vi "LIA Select Decimator.vi"(8 "error in (no error)":errorcluster, 9 "lock-in.decimator 0":enum16{"CIC", "FIR", "None"}(ring), 10 "lock-in.decimation 0":i32, 11 "LIA Host Interface in":refnum<class "LIA Host Interface.lvclass">) -> (0 "error out":errorcluster, 3 "LIA Host Interface out":refnum<class "LIA Host Interface.lvclass">)   [LabVIEW 2017]
uses:
  Program Files (x86)/National Instruments/LabVIEW 2017/examples/Lock-In Amplifier/lib/interface/Interface/LIA Host Interface.lvclass
  Program Files (x86)/National Instruments/LabVIEW 2017/examples/Lock-In Amplifier/lib/interface/Interface FPGA/LIA Host Interface FPGA.lvclass
  Program Files (x86)/National Instruments/LabVIEW 2017/examples/Lock-In Amplifier/lib/host/Public/fpga type.ctl
  Program Files (x86)/National Instruments/LabVIEW 2017/examples/Lock-In Amplifier/lib/interface/Interface FPGA/Properties/FpgaSession_GET.vi
  <vilib>/Utility/error.llb/Error Cluster From Error Code.vi
  <vilib>/rvi/errors/niLvFpgaAdjustHostInterfaceError.vi
  <vilib>/rvi/interface/nirviReadWriteControl/nirviReadWriteControl.xnode
  Program Files (x86)/National Instruments/LabVIEW 2017/examples/Lock-In Amplifier/lib/host/Lock-In Amplifier Example Host.lvlib
  NiFpgaLv.dll
  <vilib>/rvi/interface/Simulation/niFpgaSimulationCallBeginRW.vi
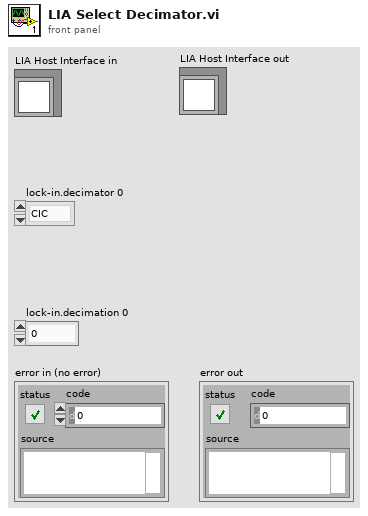
[diagram p1: front panel]
types:
  T1 = typedef "Lock-In Amplifier Example Host.lvlib/fpga type.ctl" = refnum<k20>
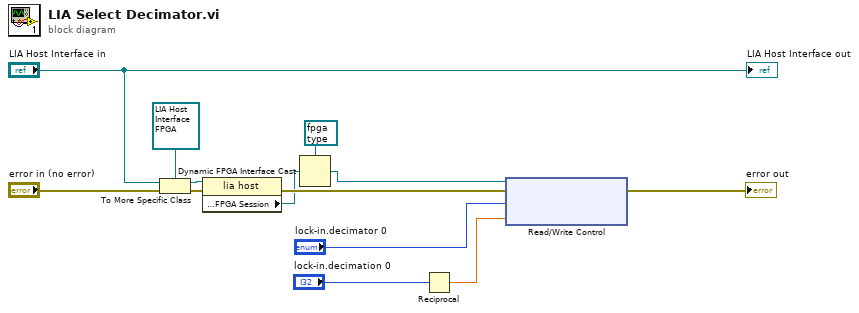
[diagram p0: block diagram]
diagram:
  n1 = To More Specific Class(target class=refnum<class "LIA Host Interface FPGA.lvclass"> refnum ("lia host"), reference="LIA Host Interface in", error in="error in (no error)") -> (specific class reference=w5:refnum<class "LIA Host Interface FPGA.lvclass">, error out=w4:errorcluster)
  n2 = property class="lia host"(reference=w5, error in=w4) -> (error out=w12:errorcluster, "Properties:FPGA Session"=w6:refnum<k20>)  [unwired: 1 out]
  n3 = Dynamic FPGA Interface Cast(Session In=T1 refnum ("fpga type"), Type=w6) -> (Session Out=w11:T1)
  n4 = Reciprocal(x="lock-in.decimation 0") -> (1/x=w10:dbl)
  n5 = xnode "Read/Write Control"("FPGA VI Reference In"=w11, "error in"=w12, "lock-in.decimator 0"="lock-in.decimator 0", "lock-in.fir fs"=w10) -> ("error out"=→"error out":errorcluster)  [unwired: 1 out]
  "LIA Host Interface out" <- "LIA Host Interface in"
